vi "Initialize FPGA (MWT) (SubVI).vi"(7 "Parameters":T1={"File REF"={"AVI REF"=refnum, "DBDE REF"=refnum}, "Frame Data"={"Width"=0, "Height"=0, "Frames Per Second"=0, "Codec"=""}, "File Type"="", "Experiment Mode"=enum."Replay", "Movie File Path"=path "D:/Movies Formatted on November 5th 2015/Clip (2) Formatted.raw"}, 8 "N Spline Points":fxp<+,8,8>=41.0, 9 "Min Contour Points":u16=127, 10 "Settings File Name":path=path "C:/MWT/Config.ini", 11 "FPGA REF (MWT) IN":T5) -> (0 "Camera OK?":bool, 3 "FPGA REF (DBDE) OUT":T5)   [LabVIEW 2020]
uses:
  Controls (HOST)/FPGA REF (MWT).ctl
  Controls (HOST)/IMAQ Parameters.ctl
  Controls (HOST)/File REF.ctl
  <vilib>/vision/Avi.llb/IMAQ AVI2 Refnum.ctl
  Controls (HOST)/Experiment Mode.ctl
  <vilib>/Utility/error.llb/Error Cluster From Error Code.vi
  <vilib>/rvi/errors/niLvFpgaAdjustHostInterfaceError.vi
  <vilib>/rvi/interface/common/niFpgaWaitOnOcc.vi
  <vilib>/FPGAPlugInAG/Dynamic/niLvFpga_Run_Dynamic.vi
  <vilib>/rvi/interface/nirviReadWriteControl/nirviReadWriteControl.xnode
  <vilib>/rvi/interface/nirviMethod/nirviMethod.xnode
  <vilib>/rvi/errors/niLvFpgaMergeErrorWithErrorCode.vi
  <vilib>/rvi/interface/Simulation/niFpgaSimulationCallBeginRW.vi
  <vilib>/FPGAPlugInAG/Dynamic/niLvFpga_ConfigureFifo_Dynamic.vi
  <vilib>/FPGAPlugInAG/Dynamic/niLvFpga_StartFifo_Dynamic.vi
  NiFpgaLv.dll
  <vilib>/FPGAPlugInAG/Dynamic/niLvFpga_WriteFifo_Dynamic.vi
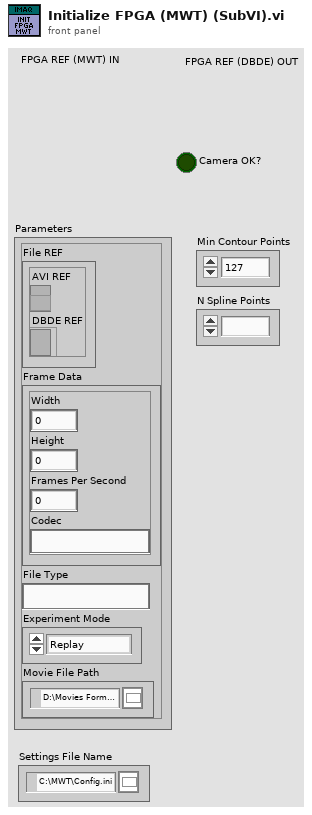
[diagram p1: front panel]
types:
  T1 = typedef "IMAQ Parameters.ctl" = cluster{"File REF":T2, "Frame Data":cluster{"Width":u32, "Height":u32, "Frames Per Second":u32, "Codec":string}, "File Type":string, "Experiment Mode":T4, "Movie File Path":path}
  T2 = typedef "File REF.ctl" = cluster{"AVI REF":T3, "DBDE REF":refnum<file>}
  T3 = typedef "IMAQ AVI2 Refnum.ctl" = refnum<k20>
  T4 = typedef "Experiment Mode.ctl" = enum16{"Live", "Replay"}
  T5 = typedef "FPGA REF (MWT).ctl" = refnum<k20>
  T6 = enum8{"Standard", "Basler 10-tap", "Vosskühler 10-tap"}
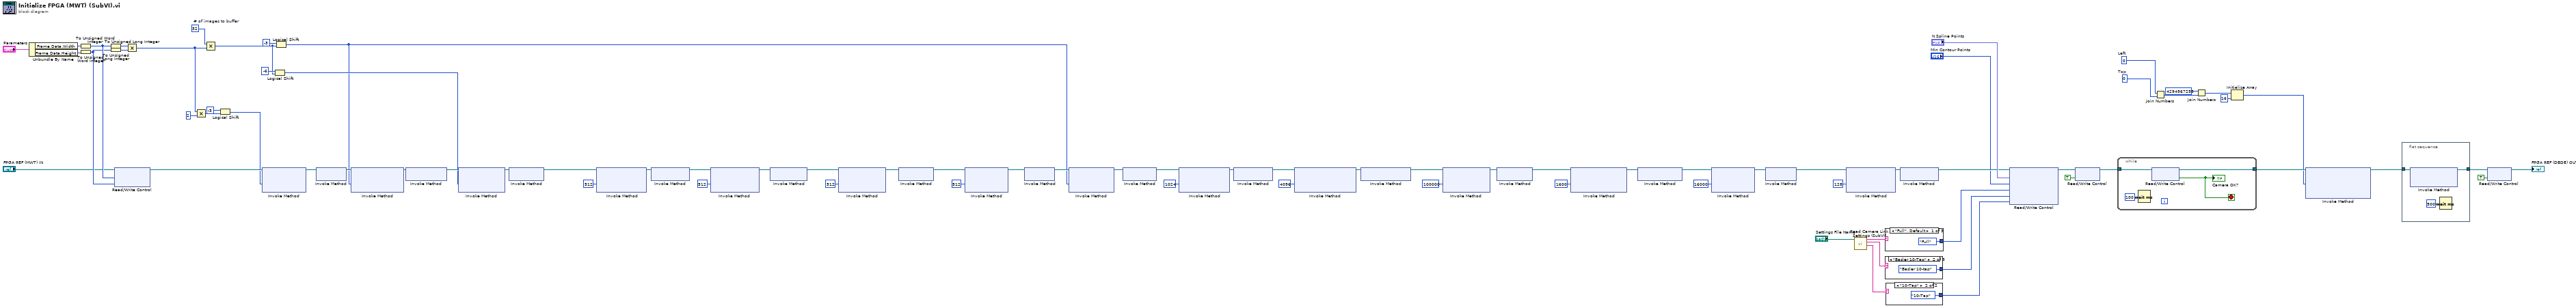
[diagram p0: block diagram]
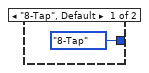
[diagram p2: hidden frame]
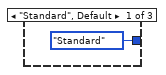
[diagram p3: hidden frame]
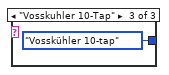
[diagram p4: hidden frame]
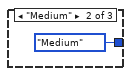
[diagram p5: hidden frame]
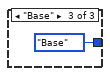
[diagram p6: hidden frame]
diagram:
  w39 = u16 0  # Top
  w42 = u16 0  # Left
  w76 = u32 32  # # of images to buffer
  n1 = Unbundle By Name("Parameters") -> ("Frame Data.Width"=w60:u32, "Frame Data.Height"=w61:u32)
  n2 = To Unsigned Word Integer(number=w60) -> (unsigned 16bit integer=w56:u16)
  n3 = To Unsigned Word Integer(number=w61) -> (unsigned 16bit integer=w55:u16)
  n4 = To Unsigned Long Integer(number=w56) -> (unsigned 32bit integer=w54:u32)
  n5 = To Unsigned Long Integer(number=w55) -> (unsigned 32bit integer=w53:u32)
  n6 = xnode "Read/Write Control"("FPGA VI Reference In"="FPGA REF (MWT) IN", "Image Width"=w56, "Image Height"=w55) -> ("FPGA VI Reference Out"=w50:T5)  [unwired: 1 in, 1 out]
  n7 = Multiply(x=w54, y=w53) -> (x*y=w74:u32)
  n8 = Multiply(x=w74, y=u32 2) -> (x*y=w69:u32)
  n9 = Multiply(x=w76, y=w74) -> (x*y=w64:u32)
  n10 = Logical Shift(y=i16 -3, x=w69) -> (x << y=w49:u32)
  n11 = xnode "Invoke Method"("FPGA VI Reference In"=w50, "Requested Depth"=w49) -> ("FPGA VI Reference Out"=w80:T5)  [unwired: 1 in, 2 out]
  n12 = Logical Shift(y=i16 -6, x=w64) -> (x << y=w63:u32)
  n13 = Logical Shift(y=i16 -3, x=w64) -> (x << y=w58:u32)
  n14 = xnode "Invoke Method"("FPGA VI Reference In"=w80) -> ("FPGA VI Reference Out"=w68:T5)  [unwired: 1 in, 1 out]
  n15 = xnode "Invoke Method"("FPGA VI Reference In"=w68, "Requested Depth"=w58) -> ("FPGA VI Reference Out"=w70:T5)  [unwired: 1 in, 2 out]
  n16 = xnode "Invoke Method"("FPGA VI Reference In"=w70) -> ("FPGA VI Reference Out"=w72:T5)  [unwired: 1 in, 1 out]
  n17 = xnode "Invoke Method"("FPGA VI Reference In"=w72, "Requested Depth"=w63) -> ("FPGA VI Reference Out"=w71:T5)  [unwired: 1 in, 2 out]
  n18 = xnode "Invoke Method"("FPGA VI Reference In"=w71) -> ("FPGA VI Reference Out"=w67:T5)  [unwired: 1 in, 1 out]
  n19 = xnode "Invoke Method"("FPGA VI Reference In"=w67, "Requested Depth"=u32 512) -> ("FPGA VI Reference Out"=w16:T5)  [unwired: 1 in, 2 out]
  n20 = xnode "Invoke Method"("FPGA VI Reference In"=w16) -> ("FPGA VI Reference Out"=w23:T5)  [unwired: 1 in, 1 out]
  n21 = xnode "Invoke Method"("FPGA VI Reference In"=w23, "Requested Depth"=u32 512) -> ("FPGA VI Reference Out"=w25:T5)  [unwired: 1 in, 2 out]
  n22 = xnode "Invoke Method"("FPGA VI Reference In"=w25) -> ("FPGA VI Reference Out"=w22:T5)  [unwired: 1 in, 1 out]
  n23 = xnode "Invoke Method"("FPGA VI Reference In"=w22, "Requested Depth"=u32 512) -> ("FPGA VI Reference Out"=w17:T5)  [unwired: 1 in, 2 out]
  n24 = xnode "Invoke Method"("FPGA VI Reference In"=w17) -> ("FPGA VI Reference Out"=w43:T5)  [unwired: 1 in, 1 out]
  n25 = xnode "Invoke Method"("FPGA VI Reference In"=w43, "Requested Depth"=u32 512) -> ("FPGA VI Reference Out"=w79:T5)  [unwired: 1 in, 2 out]
  n26 = xnode "Invoke Method"("FPGA VI Reference In"=w79) -> ("FPGA VI Reference Out"=w78:T5)  [unwired: 1 in, 1 out]
  n27 = xnode "Invoke Method"("FPGA VI Reference In"=w78, "Requested Depth"=w58) -> ("FPGA VI Reference Out"=w48:T5)  [unwired: 1 in, 2 out]
  n28 = xnode "Invoke Method"("FPGA VI Reference In"=w48) -> ("FPGA VI Reference Out"=w47:T5)  [unwired: 1 in, 1 out]
  n29 = xnode "Invoke Method"("FPGA VI Reference In"=w47, "Requested Depth"=u32 1024) -> ("FPGA VI Reference Out"=w14:T5)  [unwired: 1 in, 2 out]
  n30 = xnode "Invoke Method"("FPGA VI Reference In"=w14) -> ("FPGA VI Reference Out"=w38:T5)  [unwired: 1 in, 1 out]
  n31 = xnode "Invoke Method"("FPGA VI Reference In"=w38, "Requested Depth"=u32 4096) -> ("FPGA VI Reference Out"=w33:T5)  [unwired: 1 in, 2 out]
  n32 = xnode "Invoke Method"("FPGA VI Reference In"=w33) -> ("FPGA VI Reference Out"=w35:T5)  [unwired: 1 in, 1 out]
  n33 = xnode "Invoke Method"("FPGA VI Reference In"=w35, "Requested Depth"=u32 100000) -> ("FPGA VI Reference Out"=w34:T5)  [unwired: 1 in, 2 out]
  n34 = xnode "Invoke Method"("FPGA VI Reference In"=w34) -> ("FPGA VI Reference Out"=w27:T5)  [unwired: 1 in, 1 out]
  n35 = xnode "Invoke Method"("FPGA VI Reference In"=w27, "Requested Depth"=u32 1600) -> ("FPGA VI Reference Out"=w28:T5)  [unwired: 1 in, 2 out]
  n36 = xnode "Invoke Method"("FPGA VI Reference In"=w28) -> ("FPGA VI Reference Out"=w26:T5)  [unwired: 1 in, 1 out]
  n37 = xnode "Invoke Method"("FPGA VI Reference In"=w26, "Requested Depth"=u32 16000) -> ("FPGA VI Reference Out"=w31:T5)  [unwired: 1 in, 2 out]
  n38 = xnode "Invoke Method"("FPGA VI Reference In"=w31) -> ("FPGA VI Reference Out"=w10:T5)  [unwired: 1 in, 1 out]
  n39 = xnode "Invoke Method"("FPGA VI Reference In"=w10, "Requested Depth"=u32 128) -> ("FPGA VI Reference Out"=w11:T5)  [unwired: 1 in, 2 out]
  n40 = call "Read Camera Link Settings (SubVI).vi"("Settings File Name"="Settings File Name") -> ("Tap Configuration"=w5:string, "Signal Mapping"=w6:string, "CL Configuration"=w7:string)  [unwired: 8 in]
  n41 = case shown="\"Full\", Default" w7 {
    tunnel: [enum8{"Base", "Medium", "Full"}."Full" ("CL Config.Configuration") enum8{"Base", "Medium", "Full"}."Medium" ("CL Config.Configuration") enum8{"Base", "Medium", "Full"}."Base" ("CL Config.Configuration")] -> w4
    frame "Full", Default {
    }
    frame "Medium" {
    }
    frame "Base" {
    }
  }
  n42 = case shown="\"Basler 10-Tap\"" w6 {
    tunnel: [T6."Standard" ("CL Config.Signal Mapping") T6."Basler 10-tap" ("CL Config.Signal Mapping") T6."Vosskühler 10-tap" ("CL Config.Signal Mapping")] -> w3
    frame "Standard", Default {
    }
    frame "Basler 10-Tap" {
    }
    frame "Vosskuhler 10-Tap" {
    }
  }
  n43 = case shown="\"10-Tap\"" w5 {
    tunnel: [enum8{"8-Tap", "10-Tap"}."8-Tap" ("Tap Configuration") enum8{"8-Tap", "10-Tap"}."10-Tap" ("Tap Configuration")] -> w2
    frame "8-Tap", Default {
    }
    frame "10-Tap" {
    }
  }
  n44 = xnode "Invoke Method"("FPGA VI Reference In"=w11) -> ("FPGA VI Reference Out"=w9:T5)  [unwired: 1 in, 1 out]
  n45 = xnode "Read/Write Control"("FPGA VI Reference In"=w9, "N Spline Points"="N Spline Points", "Min Contour Points"="Min Contour Points", "Configuration"=w4, "Signal Mapping"=w3, "Tap Configuration"=w2) -> ("FPGA VI Reference Out"=w52:T5)  [unwired: 1 in, 1 out]
  n46 = xnode "Read/Write Control"("FPGA VI Reference In"=w52, "Initialize"=TRUE ("Arm Acquisition")) -> ("FPGA VI Reference Out"=w57:T5)  [unwired: 1 in, 1 out]
  n47 = while {
    tunnel: w57 -> [w94]
    tunnel: [w93] -> w45
    stop <- w91 stop-if-true
    n48 = Wait (ms)(milliseconds to wait=u32 100) -> ()  [unwired: 1 out]
    n49 = xnode "Read/Write Control"("FPGA VI Reference In"=w94) -> ("FPGA VI Reference Out"=w93:T5, "Initialized"=w91:bool)  [unwired: 1 in, 1 out]
    "Camera OK?" <- w91
  }
  n50 = Join Numbers(hi=w42, lo=w39) -> ((hi.lo)=w21:u32)
  n51 = Join Numbers(hi=u32 4294967295, lo=w21) -> ((hi.lo)=w37:u64)
  n52 = Initialize Array(w37, 16 ("dimension size")) -> (w41:u64[])
  n53 = xnode "Invoke Method"("FPGA VI Reference In"=w45, "Data"=w41) -> ("FPGA VI Reference Out"=w44:T5)  [unwired: 2 in, 2 out]
  n54 = flat-sequence {
    tunnel: w44 -> [w97]
    tunnel: [w96] -> w82
    frame #0 {
      n55 = xnode "Invoke Method"("FPGA VI Reference In"=w97) -> ("FPGA VI Reference Out"=w96:T5)  [unwired: 2 in, 1 out]
      n56 = Wait (ms)(milliseconds to wait=u32 500) -> ()  [unwired: 1 out]
    }
  }
  n57 = xnode "Read/Write Control"("FPGA VI Reference In"=w82, "Acquire"=TRUE ("Acq Control.Acquire")) -> ("FPGA VI Reference Out"=→"FPGA REF (DBDE) OUT":T5)  [unwired: 1 in, 1 out]
